vi "SPM100 control noinit v3.1.vi"(4 "error in":errorcluster, 5 "Syringe size":dbl=4.7, 6 "Pump No.":i8=3, 7 "Visa resource":refnum<visa-resource-name>="COM7") -> (0 "error out":errorcluster, 2 "dV":dbl caption="dV:" format="%#.5g", 3 "VISA resource name out":refnum<visa-resource-name>)   [LabVIEW 2014]
doc: "This is an uninitialised pump control interface for an SPM100 syringe pump. It is mainly intended for use with the CellBild imaging hardware control suite. It can however be used as a standalone interface as well if a Visa resource initialisation is performed before invoking this inteface and a Visa close action after the interface returns."
uses:
  <vilib>/Platform/TimedLoop/XDataNode/timing_clust.ctl
  <vilib>/Platform/TimedLoop/XDataNode/nitl_modes.ctl
  <vilib>/Platform/TimedLoop/XDataNode/wakeup.ctl
  <vilib>/platform/TimedLoop/XDataNode/XDataNode.xnode
  <vilib>/Platform/TimedLoop/XDataNode/XDNodeRunTimeDep.lvlib
panel:
  out "VolumeUnit 2":string="ml"
  out "FlowRateUnit disp":u32(ring) items=["ml/min", "ml/hr", "ul/min", "ul/hr"]
  out "Flow Rate disp":dbl=1.0
  out "Time run":dbl
  in  "Reset":bool
  out "return count":u32
  in  "Quit":bool
  out "Remaining time (s)":dbl=25.086956521739133 format="%.1f"
  in  "Stop":bool
  out "Remaining volume":dbl(slide)=1.0 scale=0.0..100.0 scale format="%.0f%%"
  out "Time to run (s)":dbl=26.086956521739133 format="%.1f"
  out "VolumeUnit":string="ml"
  in  "FlowRateUnit":u32(ring) items=["ml/min", "ml/hr", "ul/min", "ul/hr"]
  in  "Flow rate":dbl=1.0
  in  "Run":bool
  in  "Infuse/\nWithdraw":bool=TRUE caption="Push/Pull"
  in  "Volume":dbl=0.75
  # "SPM 100 Syringe Pump - Manual controls"
  # "Flow parameter settings"
  # "Status"
  # "Return to CellBild"
  # "Control"
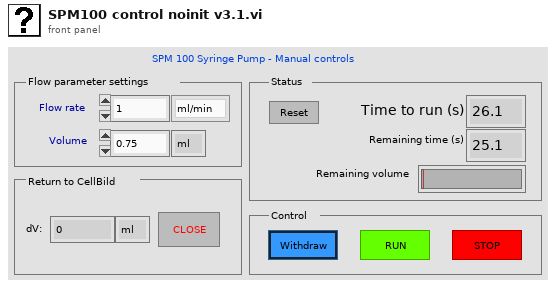
[diagram p1: front panel]
types:
  T1 = typedef "XDNodeRunTimeDep.lvlib/timing_clust.ctl" = cluster{"Expected End [f-1]":u64, "Actual End [f-1]":u64, "Finished Late? [f-1]":bool, "Expected End [i-1]":u64, "Actual End [i-1]":u64, "Finished Late? [i-1]":bool, "Expected Start [i]":u64, "Actual Start [i]":u64, "Expected Start [f]":u64, "Actual Start [f]":u64, "Source Name":string, "Structure Name":string, "Period":i64, "Deadline":i64, "Offset":i64, "Start":i64, "Priority":i32, "Timeout":i32, "Mode":T2, "Wakeup Reason":T3, "Error":errorcluster, "Source Type":string, "Secondary Source Type":string, "Global End Time":u64, "Global Start Time":u64, "Frame Duration":u64, "Iteration Duration":u64, "Assigned CPU":i32, "I/O Scan Engine Mode":u32}
  T2 = typedef "XDNodeRunTimeDep.lvlib/nitl_modes.ctl" = enum32{"No Change", "Process missed periods, maintain original phase", "Discard missed periods, maintain original phase", "Process missed periods, ignore original phase", "Discard missed periods, ignore original phase"}
  T3 = typedef "XDNodeRunTimeDep.lvlib/wakeup.ctl" = enum32{"Normal", "Aborted", "Asynchronous wakeup", "Timing source error", "Timed loop error", "Timeout"}
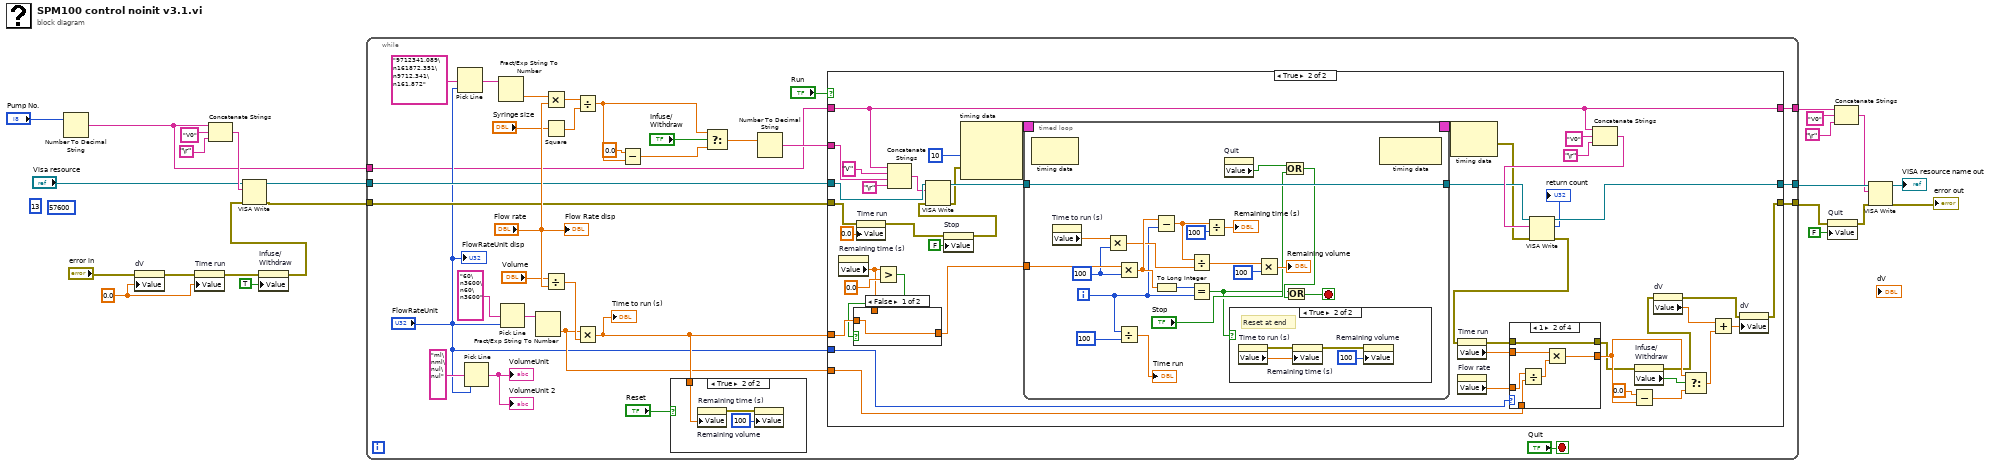
[diagram p0: block diagram]
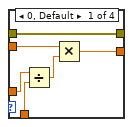
[diagram p4: hidden frame]
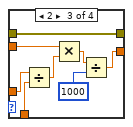
[diagram p5: hidden frame]
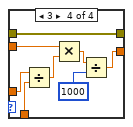
[diagram p6: hidden frame]
diagram:
  w12 = 0.0 ("dV")
  (unwired) u8 13 ("termination char\n(0xD = '\\r' = CR)")
  (unwired) u32 57600 ("baud rate")
  n1 = Number To Decimal String(number="Pump No.") -> (decimal integer string=w4:string)  [unwired: 1 in]
  n2 = property on="dV" class="DigNum (strict)"(error in="error in", "Value"=w12) -> (error out=w13:errorcluster)  [unwired: 1 in, 1 out]
  n3 = property on="Time run" class="DigNum (strict)"(error in=w13, "Value"=w12) -> (error out=w3:errorcluster)  [unwired: 1 in, 1 out]
  n4 = Concatenate Strings(w4, "V0" ("Write Command 2"), "\r") -> (w11:string)
  n5 = property on="Infuse/\nWithdraw" class="Bool (strict)"(error in=w3, "Value"=TRUE ("Infuse/\nWithdraw")) -> (error out=w2:errorcluster)  [unwired: 1 in, 1 out]
  n6 = VISA Write(VISA resource name="Visa resource", write buffer=w11, error in (no error)=w2) -> (VISA resource name out=w6:refnum<visa-resource-name>, error out=w5:errorcluster)  [unwired: 1 out]
  n7 = while {
    tunnel: [w55] -> w24
    tunnel: [w54] -> w19
    tunnel: [w35] -> w22
    tunnel: w6 -> [w30]
    tunnel: w5 -> [w29]
    tunnel: w4 -> [w26]
    stop <- "Quit" stop-if-true
    n8 = Pick Line(multi-line string="9712341.089\n161872.351\n9712.341\n161.872", line index="FlowRateUnit") -> (output string=w43:string)  [unwired: 1 in]
    n9 = Pick Line(multi-line string="ml\nml\nul\nul", line index="FlowRateUnit") -> (output string=→"VolumeUnit" →"VolumeUnit 2":string)  [unwired: 1 in]
    n10 = Fract/Exp String To Number(string=w43) -> (number=w42:dbl)  [unwired: 3 in, 1 out]
    n11 = Pick Line(multi-line string="60\n3600\n60\n3600", line index="FlowRateUnit") -> (output string=w40:string)  [unwired: 1 in]
    n12 = Fract/Exp String To Number(string=w40) -> (number=w28:dbl)  [unwired: 3 in, 1 out]
    n13 = Multiply(x=w42, y="Flow rate") -> (x*y=w53:dbl)
    n14 = Square(x="Syringe size") -> (x^2=w52:dbl)
    n15 = Divide(x="Volume", y="Flow rate") -> (x/y=w47:dbl)
    n16 = Divide(x=w53, y=w52) -> (x/y=w49:dbl)
    n17 = Multiply(x=w28, y=w47) -> (x*y=w31:dbl)
    "Time to run (s)" <- w31
    n18 = Subtract(x=0.0, y=w49) -> (x-y=w50:dbl)
    n19 = case shown="True" "Reset" {
      tunnel: w31 -> [_ w58]
      frame False {
      }
      frame True {
        n20 = property on="Remaining time (s)" class="DigNum (strict)"("Value"=w58) -> (error out=w56:errorcluster)  [unwired: 2 in, 1 out]
        n21 = property on="Remaining volume" class="Slide (strict)"(error in=w56, "Value"=100 ("Volume Remain  (%)")) -> ()  [unwired: 1 in, 2 out]
      }
    }
    n22 = Select(t=w49, s="Infuse/\nWithdraw", f=w50) -> (s? t:f=w51:dbl)
    n23 = Number To Decimal String(number=w51) -> (decimal integer string=w37:string)  [unwired: 1 in]
    n24 = case shown="True" "Run" {
      tunnel: w30 -> [w61 w106]
      tunnel: w29 -> [w60 w71]
      tunnel: [w61 w96] -> w55
      tunnel: [w60 w64] -> w54
      tunnel: w31 -> [_ w94]
      tunnel: w26 -> [w59 w95]
      tunnel: w37 -> [_ w103]
      tunnel: [w59 w95] -> w35
      tunnel: w28 -> [_ w78]
      tunnel: "FlowRateUnit" -> [_ w72]
      frame False {
      }
      frame True {
        n25 = property on="Remaining time (s)" class="DigNum (strict)"() -> ("Value"=w91:dbl)  [unwired: 2 in, 2 out]
        n26 = property on="Time run" class="DigNum (strict)"(error in=w71, "Value"=0.0 ("Time run")) -> (error out=w63:errorcluster)  [unwired: 1 in, 1 out]
        n27 = Greater?(x=w91, y=0.0) -> (0:w92:bool)
        n28 = case shown="False" w92 {
          tunnel: w94 -> [w168 _]
          tunnel: [w168 w169] -> w90
          tunnel: w91 -> [_ w169]
          frame False {
          }
          frame True {
          }
        }
        n29 = Concatenate Strings(w95, "V" ("string"), w103, "\r") -> (w104:string)
        n30 = property on="Stop" class="Bool (strict)"(error in=w63, "Value"=FALSE ("Stop")) -> (error out=w62:errorcluster)  [unwired: 1 in, 1 out]
        n31 = VISA Write(VISA resource name=w106, write buffer=w104, error in (no error)=w62) -> (VISA resource name out=w105:refnum<visa-resource-name>, error out=w85:errorcluster)  [unwired: 1 out]
        n32 = node-c288(u32 10 ("millisecond multiple"), w85) -> (w87:T1)  [unwired: 1 in]
        n33 = timed-loop {
          tunnel: [w155] -> w97
          tunnel: w105 -> [w155]
          tunnel: w90 -> [w150]
          timing: w87 -> [_]
          timing-out: [_] -> w86
          i -> [w135]
          stop <- w143 stop-if-true
          w139 = 100
          n34 = node-c288() -> ()  [unwired: 1 in, 1 out]
          n35 = property on="Time to run (s)" class="DigNum (strict)"() -> ("Value"=w140:dbl)  [unwired: 2 in, 2 out]
          n36 = Multiply(x=w140, y=w139) -> (x*y=w138:dbl)
          n37 = Multiply(x=w150, y=w139) -> (x*y=w149:dbl)
          n38 = Divide(x=w135, y=100) -> (x/y=→"Time run":dbl)
          n39 = Subtract(x=w149, y=w135) -> (x-y=w153:dbl)
          n40 = To Long Integer(number=w149) -> (32bit integer=w151:i32)
          n41 = Divide(x=w153, y=w138) -> (x/y=w146:dbl)
          n42 = Equal?(x=w151, y=w135) -> (x = y?=w141:bool)
          n43 = Divide(x=w153, y=100) -> (x/y=→"Remaining time (s)":dbl)
          n44 = property on="Quit" class="Bool (strict)"() -> ("Value"=w145:bool)  [unwired: 2 in, 2 out]
          n45 = case shown="True" w141 {
            frame False {
            }
            frame True {
              # "Reset at end"
              n46 = property on="Time to run (s)" class="DigNum (strict)"() -> (error out=w159:errorcluster, "Value"=w158:dbl)  [unwired: 2 in, 1 out]
              n47 = property on="Remaining time (s)" class="DigNum (strict)"(error in=w159, "Value"=w158) -> (error out=w157:errorcluster)  [unwired: 1 in, 1 out]
              n48 = property on="Remaining volume" class="Slide (strict)"(error in=w157, "Value"=100 ("Volume Remain  (%)")) -> ()  [unwired: 1 in, 2 out]
            }
          }
          n49 = Multiply(x=w146, y=100) -> (x*y=→"Remaining volume":dbl)
          n50 = Or(x=w145, y="Stop") -> (x .or. y?=w144:bool)
          n51 = Or(x=w141, y=w144) -> (x .or. y?=w143:bool)
          n52 = node-c288() -> ()  [unwired: 1 in, 1 out]
        }
        n53 = node-c288(w86) -> (w83:errorcluster)
        n54 = property on="Flow rate" class="DigNum (strict)"() -> ("Value"=w77:dbl)  [unwired: 2 in, 2 out]
        n55 = Concatenate Strings(w95, "V0" ("Write Command 2"), "\r") -> (w98:string)
        n56 = VISA Write(VISA resource name=w97, write buffer=w98, error in (no error)=w83) -> (VISA resource name out=w96:refnum<visa-resource-name>, return count=→"return count":u32, error out=w69:errorcluster)
        n57 = property on="Time run" class="DigNum (strict)"(error in=w69) -> (error out=w68:errorcluster, "Value"=w76:dbl)  [unwired: 1 in, 1 out]
        n58 = case shown="1" w72 {
          tunnel: w78 -> [w109 w118 w126 w134]
          tunnel: w77 -> [w110 w117 w125 w133]
          tunnel: w76 -> [w111 w116 w124 w132]
          tunnel: [w108 w114 w123 w131] -> w75
          tunnel: w68 -> [w107 w113 w119 w127]
          tunnel: [w107 w113 w119 w127] -> w67
          frame 0, Default {
            n59 = Divide(x=w110, y=w109) -> (x/y=w112:dbl)
            n60 = Multiply(x=w111, y=w112) -> (x*y=w108:dbl)
          }
          frame 1 {
            n61 = Divide(x=w117, y=w118) -> (x/y=w115:dbl)
            n62 = Multiply(x=w116, y=w115) -> (x*y=w114:dbl)
          }
          frame 2 {
            n63 = Divide(x=w125, y=w126) -> (x/y=w121:dbl)
            n64 = Multiply(x=w124, y=w121) -> (x*y=w122:dbl)
            n65 = Divide(x=w122, y=1000) -> (x/y=w123:dbl)
          }
          frame 3 {
            n66 = Divide(x=w133, y=w134) -> (x/y=w129:dbl)
            n67 = Multiply(x=w132, y=w129) -> (x*y=w130:dbl)
            n68 = Divide(x=w130, y=1000) -> (x/y=w131:dbl)
          }
        }
        n69 = Subtract(x=0.0, y=w75) -> (x-y=w82:dbl)
        n70 = property on="Infuse/\nWithdraw" class="Bool (strict)"(error in=w67) -> (error out=w66:errorcluster, "Value"=w74:bool)  [unwired: 1 in, 1 out]
        n71 = property on="dV" class="DigNum (strict)"(error in=w66) -> (error out=w65:errorcluster, "Value"=w79:dbl)  [unwired: 1 in, 1 out]
        n72 = Select(t=w75, s=w74, f=w82) -> (s? t:f=w73:dbl)
        n73 = Add(x=w79, y=w73) -> (x+y=w80:dbl)
        n74 = property on="dV" class="DigNum (strict)"(error in=w65, "Value"=w80) -> (error out=w64:errorcluster)  [unwired: 1 in, 1 out]
      }
    }
    "Flow Rate disp" <- "Flow rate"
    "FlowRateUnit disp" <- "FlowRateUnit"
  }
  n75 = property on="Quit" class="Bool (strict)"(error in=w19, "Value"=FALSE ("Quit")) -> (error out=w18:errorcluster)  [unwired: 1 in, 1 out]
  n76 = Concatenate Strings(w22, "V0" ("Write Command 2"), "\r") -> (w23:string)
  n77 = VISA Write(VISA resource name=w24, write buffer=w23, error in (no error)=w18) -> (VISA resource name out=→"VISA resource name out":refnum<visa-resource-name>, error out=→"error out":errorcluster)  [unwired: 1 out]
